vi "PP_Profile_Block_Av.vi"() -> ()   [LabVIEW 2011]
panel:
  in  "Results file":path
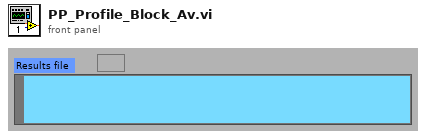
[diagram p1: front panel]
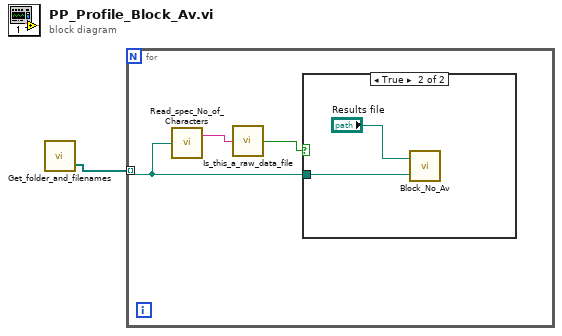
[diagram p0: block diagram]
diagram:
  n1 = call "Get_folder_and_filenames.vi"() -> ("Files"=w1:path[])  [unwired: 1 in, 1 out]
  n2 = for {
    tunnel: w1 -> [w4] mode=indexing
    n3 = call "Read_spec_No_of_Characters.vi"("Filename"=w4) -> ("character string"=w3:string)  [unwired: 1 out]
    n4 = call "Is_this_a_raw_data_file.vi"("character string"=w3) -> ("Raw Dat File?"=w2:bool)  [unwired: 2 out]
    n5 = case shown="True" w2 {
      tunnel: w4 -> [_ w5]
      frame False {
      }
      frame True {
        n6 = call "Block_No_Av.vi"("Raw data file"=w5, "Results file"="Results file") -> ()  [unwired: 2 out]
      }
    }
  }
